vi "main 2021 12 15.vi"() -> ()   [LabVIEW 2019]
panel:
  out "error out":errorcluster
  in  "error in (no error)":errorcluster
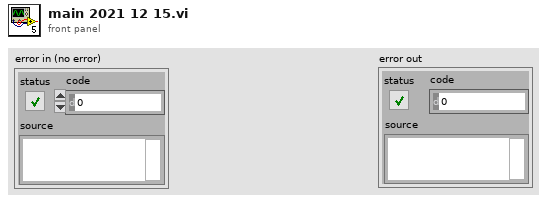
[diagram p1: front panel]
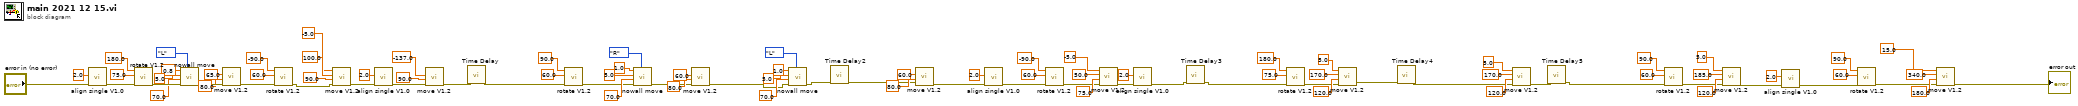
[diagram p0: block diagram]
diagram:
  n1 = call "align single V1.0.vi"("error in (no error)"="error in (no error)", "Target (Volt)"=2.0) -> ("error out"=w86:errorcluster)  [unwired: 9 in]
  n2 = call "rotate V1.2.vi"("error in (no error)"=w86, "speed"=75.0, "degree"=180.0) -> ("error out"=w83:errorcluster)  [unwired: 8 in]
  n3 = call "nowall move.vi"("dir"=enum16{"R", "L"}."L", "error in (no error)"=w83, "Speed"=70.0, "Distance"=5.0, "IR if?"=0.8) -> ("error out"=w78:errorcluster)  [unwired: 6 in]
  n4 = call "move V1.2.vi"("error in (no error)"=w78, "RPM"=80.0, "Y"=65.0) -> ("error out"=w23:errorcluster)  [unwired: 8 in]
  n5 = call "rotate V1.2.vi"("error in (no error)"=w23, "speed"=60.0, "degree"=-90.0) -> ("error out"=w3:errorcluster)  [unwired: 8 in]
  n6 = call "move V1.2.vi"("error in (no error)"=w3, "RPM"=90.0, "Y"=100.0, "X"=-5.0) -> ("error out"=w4:errorcluster)  [unwired: 7 in]
  n7 = call "align single V1.0.vi"("error in (no error)"=w4, "Target (Volt)"=2.0) -> ("error out"=w20:errorcluster)  [unwired: 9 in]
  n8 = call "move V1.2.vi"("error in (no error)"=w20, "RPM"=90.0, "Y"=-137.0) -> ("error out"=w17:errorcluster)  [unwired: 8 in]
  n9 = call "Time Delay"("error in (no error)"=w17) -> ("error out"=w15:errorcluster)  [unwired: 10 in]
  n10 = call "rotate V1.2.vi"("error in (no error)"=w15, "speed"=60.0, "degree"=90.0) -> ("error out"=w16:errorcluster)  [unwired: 8 in]
  n11 = call "nowall move.vi"("dir"=enum16{"R", "L"}."R", "error in (no error)"=w16, "Speed"=70.0, "Distance"=5.0, "IR if?"=1.0) -> ("error out"=w73:errorcluster)  [unwired: 6 in]
  n12 = call "move V1.2.vi"("error in (no error)"=w73, "RPM"=80.0, "Y"=60.0) -> ("error out"=w62:errorcluster)  [unwired: 8 in]
  n13 = call "nowall move.vi"("dir"=enum16{"R", "L"}."L", "error in (no error)"=w62, "Speed"=70.0, "Distance"=5.0, "IR if?"=1.0) -> ("error out"=w14:errorcluster)  [unwired: 6 in]
  n14 = call "Time Delay2"("error in (no error)"=w14) -> ("error out"=w13:errorcluster)  [unwired: 10 in]
  n15 = call "move V1.2.vi"("error in (no error)"=w13, "RPM"=80.0, "Y"=60.0) -> ("error out"=w60:errorcluster)  [unwired: 8 in]
  n16 = call "align single V1.0.vi"("error in (no error)"=w60, "Target (Volt)"=2.0) -> ("error out"=w57:errorcluster)  [unwired: 9 in]
  n17 = call "rotate V1.2.vi"("error in (no error)"=w57, "speed"=60.0, "degree"=-90.0) -> ("error out"=w38:errorcluster)  [unwired: 8 in]
  n18 = call "move V1.2.vi"("error in (no error)"=w38, "RPM"=75.0, "Y"=50.0, "X"=-5.0) -> ("error out"=w30:errorcluster)  [unwired: 7 in]
  n19 = call "align single V1.0.vi"("error in (no error)"=w30, "Target (Volt)"=2.0) -> ("error out"=w12:errorcluster)  [unwired: 9 in]
  n20 = call "Time Delay3"("error in (no error)"=w12) -> ("error out"=w11:errorcluster)  [unwired: 10 in]
  n21 = call "rotate V1.2.vi"("error in (no error)"=w11, "speed"=75.0, "degree"=180.0) -> ("error out"=w52:errorcluster)  [unwired: 8 in]
  n22 = call "move V1.2.vi"("error in (no error)"=w52, "RPM"=120.0, "Y"=170.0, "X"=5.0) -> ("error out"=w10:errorcluster)  [unwired: 7 in]
  n23 = call "Time Delay4"("error in (no error)"=w10) -> ("error out"=w9:errorcluster)  [unwired: 10 in]
  n24 = call "move V1.2.vi"("error in (no error)"=w9, "RPM"=120.0, "Y"=170.0, "X"=5.0) -> ("error out"=w8:errorcluster)  [unwired: 7 in]
  n25 = call "Time Delay5"("error in (no error)"=w8) -> ("error out"=w7:errorcluster)  [unwired: 10 in]
  n26 = call "rotate V1.2.vi"("error in (no error)"=w7, "speed"=60.0, "degree"=90.0) -> ("error out"=w47:errorcluster)  [unwired: 8 in]
  n27 = call "move V1.2.vi"("error in (no error)"=w47, "RPM"=120.0, "Y"=185.0, "X"=5.0) -> ("error out"=w36:errorcluster)  [unwired: 7 in]
  n28 = call "align single V1.0.vi"("error in (no error)"=w36, "Target (Volt)"=2.0) -> ("error out"=w35:errorcluster)  [unwired: 9 in]
  n29 = call "rotate V1.2.vi"("error in (no error)"=w35, "speed"=60.0, "degree"=90.0) -> ("error out"=w42:errorcluster)  [unwired: 8 in]
  n30 = call "move V1.2.vi"("error in (no error)"=w42, "RPM"=180.0, "Y"=340.0, "X"=15.0) -> ("error out"=→"error out":errorcluster)  [unwired: 7 in]
